vi "calculate_Rest.vi"(1 "wGyro":u8, 2 "Rgyro":dbl[](array[numeric]), 3 "Accelerometer readings":i32[](array[numeric])) -> (0 "Rest":dbl[](array[numeric]))   [LabVIEW 2015]
doc: "Caclulatest the estimated gravity vector using the combined readings from gyroscope and accelerometer."
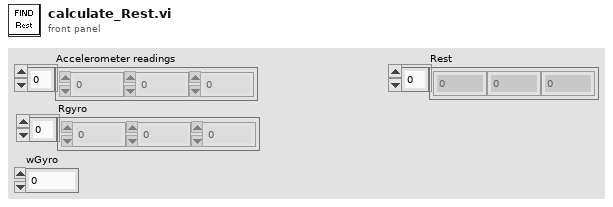
[diagram p1: front panel]
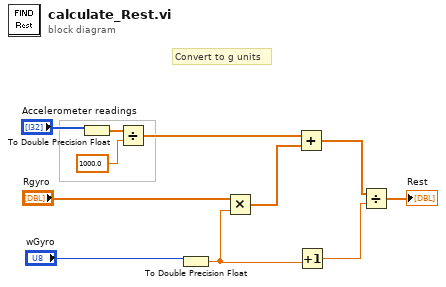
[diagram p0: block diagram]
diagram:
  # "Convert to g units"
  n1 = To Double Precision Float(number="Accelerometer readings") -> (double precision float=w7:dbl[])
  n2 = Divide(x=w7, y=1000.0) -> (x/y=w2:dbl[])
  n3 = To Double Precision Float(number="wGyro") -> (double precision float=w6:dbl)
  n4 = Multiply(x="Rgyro", y=w6) -> (x*y=w8:dbl[])
  n5 = Add(x=w2, y=w8) -> (x+y=w5:dbl[])
  n6 = Increment(x=w6) -> (x+1=w4:dbl)
  n7 = Divide(x=w5, y=w4) -> (x/y=→"Rest":dbl[])
